vi "get_histogram.vi"(8 "error in (no error)":errorcluster, 11 "DisplayDL090216 in":refnum<class "DisplayDL090216.lvclass">) -> (0 "error out":errorcluster, 2 "histogram out":cluster{i32, u32}[](graph), 3 "DisplayDL090216 out":refnum<class "DisplayDL090216.lvclass">)   [LabVIEW 2010]
uses:
  common/classes/Image/Image/Image.lvclass
  DisplayDL090216.lvclass
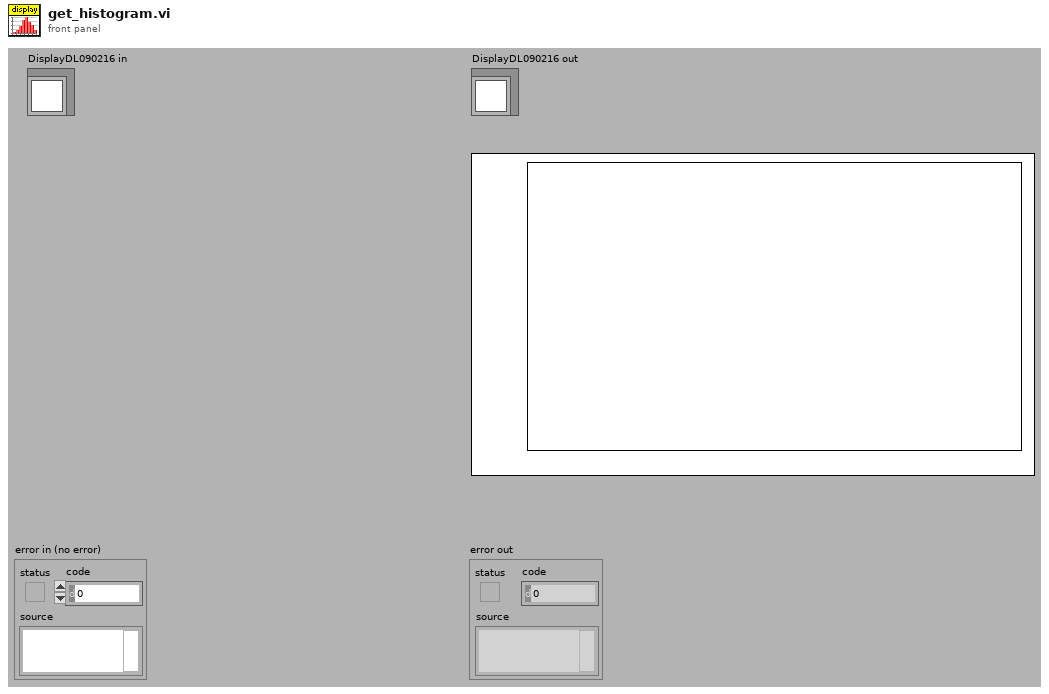
[diagram p1: front panel]
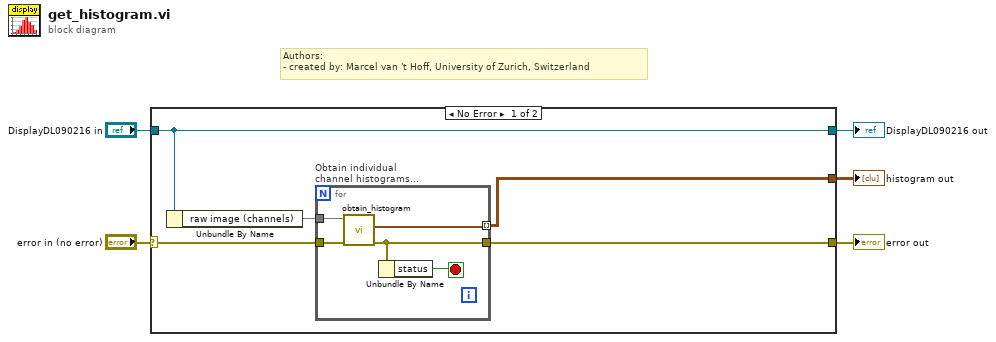
[diagram p0: block diagram]
diagram:
  # "Authors: \n- created by: Marcel van 't Hoff, University of Zurich, Switzerland"
  n1 = case shown="No Error" "error in (no error)" {
    selector: "error in (no error)" -> [w9 w17]
    tunnel: [w6 w17] -> w4
    tunnel: [w10 w16] -> w2
    tunnel: "DisplayDL090216 in" -> [w10 w16]
    tunnel: [w7 _] -> w1
    frame No Error {
      n2 = Unbundle By Name(w10) -> ("raw image (channels)"=w8)
      n3 = for "Obtain individual channel histograms..." {
        tunnel: w8 -> [w12]
        tunnel: w9 -> [w15]
        tunnel: [w14] -> w6
        tunnel: [w11] -> w7 mode=indexing
        stop <- w13 stop-if-true
        n4 = call "obtain_histogram.vi"("error in (no error)"=w15, "Image in"=w12) -> ("error out"=w14:errorcluster, "histogram out"=w11:cluster{i32, u32}[])  [unwired: 7 in, 1 out]
        n5 = Unbundle By Name(w14) -> ("status"=w13:bool)
      }
    }
    frame Error {
    }
  }
  "error out" <- w4
  "DisplayDL090216 out" <- w2
  "histogram out" <- w1
